vi "N25_Filter.vi"(11 "input data":fxp<+/-,21,1>) -> (3 "output data":fxp<+/-,21,1> format="%.31g")   [LabVIEW 2019]
doc: "----------------------\n\nThis filter is configured as follows:\n\n<b>Filter Configuration</b>\nType: Single Rate\nStructure: MA\n\n<b>Input Data Type</b>\nType: fixed-point <±,21,1> [-1,000000E+0,9,999990E-1]:9,536743E-7\n\n<b>Output Data Type</b>\nType: fixed-point <±,21,1> [-1,000000E+0,9,999990E-1]:9,536743E-7\nRounding mode: Round-Half-Even\nOverflow mode: Saturate\n\n<b>Implementation</b>\nNumber of channels: 1\nMaximum input sampling rate per channel @ 40MHz: 20MHz\nGain processing: On Host\n\n<b>Execution Mode</b>\nOutside single-cycle Timed Loop\nThroughput: 2 cycles/call"
uses:
  <vilib>/Platform/TimedLoop/XDataNode/timing_clust.ctl
  <vilib>/Platform/TimedLoop/XDataNode/nitl_modes.ctl
  <vilib>/Platform/TimedLoop/XDataNode/wakeup.ctl
  <vilib>/rvi/Emulation/niFpgaSctlEmulationGetInTimedLoop.vi
  <vilib>/rvi/Emulation/niFpgaEmulationReportErrorSimple.vi
  <vilib>/rvi/Emulation/niFpgaGetClockAttributes.vi
  <vilib>/rvi/Emulation/niFpgaCriticalErrorInLSC.vi
  <vilib>/platform/TimedLoop/XDataNode/XDataNode.xnode
  <vilib>/Platform/TimedLoop/XDataNode/XDNodeRunTimeDep.lvlib
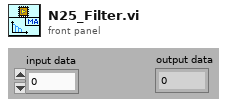
[diagram p1: front panel]
types:
  T1 = typedef "XDNodeRunTimeDep.lvlib/timing_clust.ctl" = cluster{"Expected End [f-1]":u64, "Actual End [f-1]":u64, "Finished Late? [f-1]":bool, "Expected End [i-1]":u64, "Actual End [i-1]":u64, "Finished Late? [i-1]":bool, "Expected Start [i]":u64, "Actual Start [i]":u64, "Expected Start [f]":u64, "Actual Start [f]":u64, "Source Name":string, "Structure Name":string, "Period":i64, "Deadline":i64, "Offset":i64, "Start":i64, "Priority":i32, "Timeout":i32, "Mode":T2, "Wakeup Reason":T3, "Error":errorcluster, "Source Type":string, "Secondary Source Type":string, "Global End Time":u64, "Global Start Time":u64, "Frame Duration":u64, "Iteration Duration":u64, "Assigned CPU":i32, "I/O Scan Engine Mode":u32}
  T2 = typedef "XDNodeRunTimeDep.lvlib/nitl_modes.ctl" = enum32{"No Change", "Process missed periods, maintain original phase", "Discard missed periods, maintain original phase", "Process missed periods, ignore original phase", "Discard missed periods, ignore original phase"}
  T3 = typedef "XDNodeRunTimeDep.lvlib/wakeup.ctl" = enum32{"Normal", "Aborted", "Asynchronous wakeup", "Timing source error", "Timed loop error", "Timeout"}
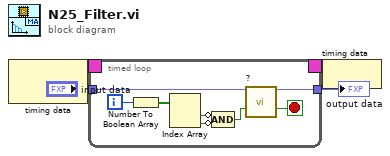
[diagram p0: block diagram]
diagram:
  n1 = node-c288() -> (w2:T1)  [unwired: 1 in]
  n2 = timed-loop "Main While Loop" {
    tunnel: [w11] -> w4
    tunnel: "input data" -> [w10]
    timing: w2 -> [_]
    timing-out: [_] -> w1
    i -> [w9]
    stop <- w12 stop-if-true
    n3 = Number To Boolean Array(number=w9) -> (Boolean array=w8:bool[])
    n4 = Index Array(array=w8) -> (element #1=w7:bool, element #2=w6:bool)  [unwired: 2 in]
    n5 = Compound Arithmetic op=AND(invert w7, invert w6) -> (w5:bool)
    n6 = call "?"("input data"=w10, "input valid"=w5) -> ("output data"=w11:fxp<+/-,21,1>, "output valid"=w12:bool)  [unwired: 11 in, 1 out]
  }
  "output data" <- w4
  n7 = node-c288(w1) -> ()
